vi "Read Message (TCP).vi"(6 "options":T2={"ignore timeout error"=TRUE, "timeout ms (1000)"=1000}, 8 "error in":errorcluster, 11 "connection info in":T4) -> (0 "error out":errorcluster, 1 "name":T3, 2 "data string":string, 3 "connection info out":T4, 4 "data info":T1, 5 "timed out?":bool)   [LabVIEW 2010, in "NI STM.lvlib"]
doc: "This VI reads an incoming package of data from a host. This VI parses the package and extracts the data name and type as described in the meta data.\n\nFor the package to be parsed correctly, the meta data must be consistent in both the sender and the receiver. The data is packaged based on the existing meta data on the sender. \n\nUse the \"STM Read Meta Data\" and \"STM Write Meta Data\" VIs to ensure that both client and server have the same meta data.\n\nThe data is returned as a string. It is the responsibility of the user to cast it to the appropriate type.\n\nCopyright 2015, 2016, 2017 National Instruments Corporation\n\nLicensed under the Apache License, Version 2.0 (the \"License\"); you may not use this file except in compliance with the License.\n\n You may obtain a copy of the License at\n\n http://www.apache.org/licenses/LICENSE-2.0\n\nUnless required by applicable law or agreed to in writing, software distributed under the License is distributed on an \"AS IS\" BASIS, WITHOUT WARRANTIES OR CONDITIONS OF ANY KIND, either express or implied.\n\nSee the License for the specific language governing permissions and limitations under the License."
uses:
  NI STM.lvlib
  TCP Connection Info.ctl
  SubVIs/MetaDataElement.ctl
  TCP Read Options.ctl
  TCP Data Info.ctl
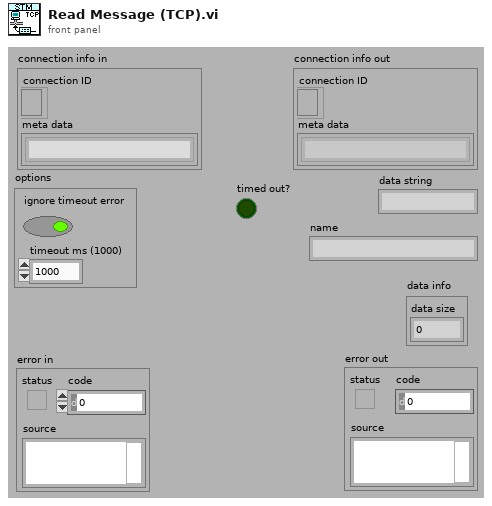
[diagram p1: front panel]
types:
  T1 = typedef "NI STM.lvlib/TCP Data Info.ctl" = cluster{"data size":i32}
  T2 = typedef "NI STM.lvlib/TCP Read Options.ctl" = cluster{"ignore timeout error":bool, "timeout ms (1000)":i32}
  T3 = typedef "NI STM.lvlib/MetaDataElement.ctl" = string
  T4 = typedef "NI STM.lvlib/TCP Connection Info.ctl" = cluster{"connection ID":refnum<k5>, "meta data":T3[]}
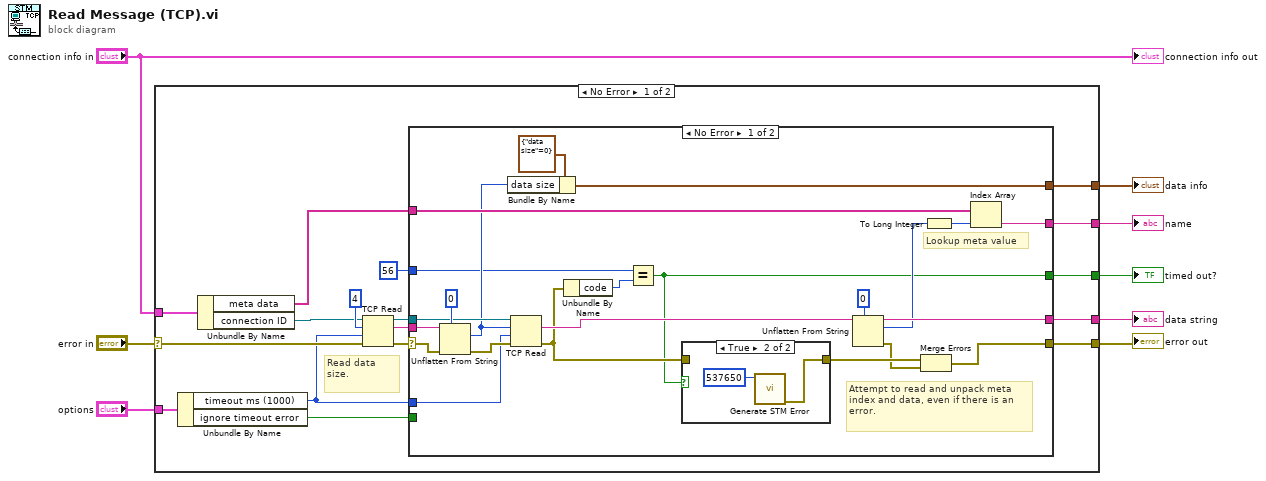
[diagram p0: block diagram]
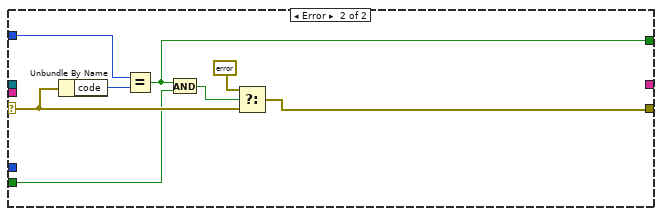
[diagram p3: hidden frame]
diagram:
  n1 = case shown="No Error" "error in" {
    selector: "error in" -> [w12 w60]
    tunnel: "connection info in" -> [w11 _]
    tunnel: [w21 w60] -> w8
    tunnel: [w20 _] -> w7
    tunnel: [w19 _] -> w6
    tunnel: [w18 _] -> w5
    tunnel: [w17 _] -> w2
    tunnel: "options" -> [w13 _]
    frame No Error {
      # "Read data size."
      n2 = Unbundle By Name(w13) -> ("timeout ms (1000)"=w10:i32, "ignore timeout error"=w16:bool)
      n3 = Unbundle By Name(w11) -> ("meta data"=w14:T3[], "connection ID"=w15:refnum<k5>)
      n4 = TCP Read(connection ID=w15, bytes to read=4, error in (no error)=w12, 9:w10) -> (connection ID out=w23:refnum<k5>, data out=w24:string, error out=w22:errorcluster)  [unwired: 1 out]
      n5 = case shown="No Error" w22 {
        selector: w22 -> [w44 w59]
        tunnel: w24 -> [w45 _]
        tunnel: w23 -> [w47 _]
        tunnel: w14 -> [w46 _]
        tunnel: [w26 w58] -> w21
        tunnel: w16 -> [_ w55]
        tunnel: [w29 w52] -> w20
        tunnel: [w43 _] -> w19
        tunnel: [w39 _] -> w18
        tunnel: [w32 _] -> w17
        tunnel: w10 -> [w35 _]
        tunnel: 56 ("code") -> [w31 w57]
        frame No Error {
          # "Lookup meta value"
          # "Attempt to read and unpack meta index and data, even if there is an error."
          n6 = Unflatten From String(type=0 ("bytes to read"), binary string=w45, error in (no error)=w44) -> (value=w33:i32, error out=w41:errorcluster)  [unwired: 1 in, 2 out]
          n7 = Bundle By Name(cluster=T1 {"data size"=0} ("Data Info"), "data size"=w33) -> (w32:T1)
          n8 = TCP Read(connection ID=w47, bytes to read=w33, error in (no error)=w41, 9:w35) -> (data out=w42:string, error out=w36:errorcluster)  [unwired: 2 out]
          n9 = Unbundle By Name(w36) -> ("code"=w30:i32)
          n10 = Equal?(x=w31, y=w30) -> (x = y?=w29:bool)
          n11 = case shown="True" w29 {
            tunnel: w36 -> [w49 _]
            tunnel: [w49 w50] -> w28
            frame False {
            }
            frame True {
              n12 = call "Generate STM Error.vi"("code"=537650) -> ("error out"=w50:errorcluster)  [unwired: 10 in]
            }
          }
          n13 = Unflatten From String(type=u16 0 ("bytes to read"), binary string=w42) -> (rest of the binary string=w39:string, value=w37:u16, error out=w27:errorcluster)  [unwired: 1 in, 2 out]
          n14 = Merge Errors(w28, w27) -> (w26:errorcluster)
          n15 = To Long Integer(number=w37) -> (32bit integer=w38:i32)
          n16 = Index Array(array=w46, index=w38) -> (element=w43:T3)
        }
        frame Error {
          n17 = Unbundle By Name(w59) -> ("code"=w56:i32)
          n18 = Equal?(x=w57, y=w56) -> (x = y?=w52:bool)
          n19 = And(x=w52, y=w55) -> (x .and. y?=w54:bool)
          n20 = Select(t=errorcluster {"status"=FALSE, "code"=0, "source"=""} ("error out"), s=w54, f=w59) -> (s? t:f=w58:errorcluster)
        }
      }
    }
    frame Error {
    }
  }
  "error out" <- w8
  "timed out?" <- w7
  "data string" <- w5
  "name" <- w6
  "data info" <- w2
  "connection info out" <- "connection info in"
